vi "SpectrumCursor_write.vi"(1 "cursor position":cluster{"X":dbl, "Y":dbl}, 2 "existing\ncursor name":string="poly", 3 "graph ref":refnum<vi>) -> ()   [LabVIEW 2010]
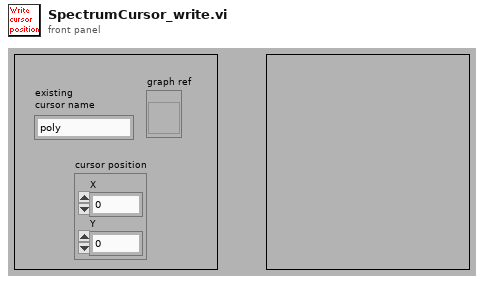
[diagram p1: front panel]
types:
  T1 = typedef "LVCursorListTypeDef.ctl" = cluster{"Name":string, "Color":u32, "Style":u8, "Point Style":u8, "Name Visible":bool, "Allow Drag":bool, "Cursor Mode":u32, "Plot":i32, "Index":i32, "Position":cluster{"X":dbl, "Y":dbl}, "X Scale":u32, "Y Scale":u32, "Watch Plots":i32[], "Watch All Plots":bool, "Plot Area":i32, "Label Offset":cluster{"X":dbl, "Y":dbl}}[]
  T2 = cluster{"Name":string, "Color":u32, "Style":u8, "Point Style":u8, "Name Visible":bool, "Allow Drag":bool, "Cursor Mode":u32, "Plot":i32, "Index":i32, "Position":cluster{"X":dbl, "Y":dbl}, "X Scale":u32, "Y Scale":u32, "Watch Plots":i32[], "Watch All Plots":bool, "Plot Area":i32, "Label Offset":cluster{"X":dbl, "Y":dbl}}
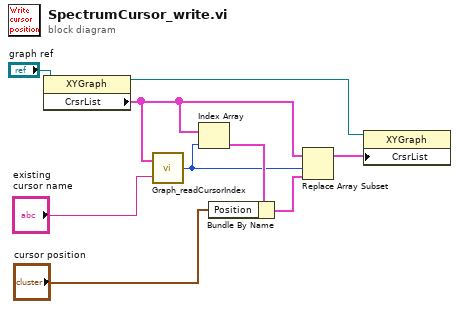
[diagram p0: block diagram]
diagram:
  n1 = property class="XYGraph"(reference="graph ref") -> (reference out=w2:refnum<vi>, "CrsrList"=w4:T1)  [unwired: 1 in, 1 out]
  n2 = call "Graph_readCursorIndex.vi"("existing cursor\nname"="existing\ncursor name", "Cursor List"=w4) -> ("cursor index"=w5:i32)
  n3 = Index Array(array=w4, index=w5) -> (element=w7:T2)
  n4 = Bundle By Name(cluster=w7, "Position"="cursor position") -> (w3:T2)
  n5 = Replace Array Subset(array=w4, new element=w3, index=w5) -> (w1:T1)
  n6 = property class="XYGraph"(reference=w2, "CrsrList"=w1) -> ()  [unwired: 1 in, 2 out]
